vi "CRYPlot Result.vi"(7 "pGraph VI In":refnum<vi>, 8 "Graph Set?":bool, 9 "Flattened Property":string, 10 "New Rows In":i32[](array[numeric]), 11 "Old Rows In":i32[](array[numeric])) -> (2 "Curve Name":string[](array[string]), 3 "Selected Rows Out":i32[](array[numeric]))   [LabVIEW 2013]
uses:
  CRYWindow/DataView/Control/CRYResult Property.ctl
panel:
  in  "Result Property":T1={"Show Limits"=FALSE, "Show Yield"=FALSE, "Pass/Fail"=FALSE, "Notation"=0, "Digits"=0, "Precision"=0, "Hide Traling Zeros"=FALSE, "Show vertical scroll bar"=FALSE, "Show horizontal scroll bar"=FALSE, "True"="NO ELECTRICAL SIGNAL DETECTED!\nCheck wiring and connections.", "False"="NO ELECTRICAL SIGNAL DETECTED!\nCheck wiring and connections.", "Font Size"=0, "Overall/Optional"=0} {"Precision" items=["Digits of precision", "Significant digits"]}
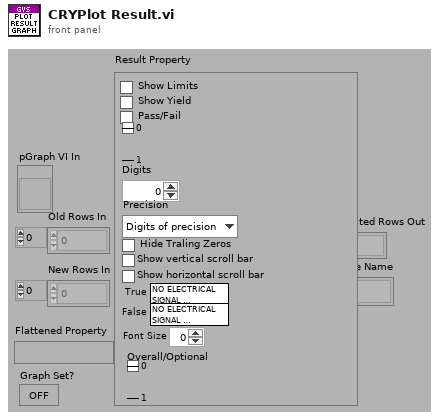
[diagram p1: front panel]
types:
  T1 = typedef "CRYResult Property.ctl" = cluster{"Show Limits":bool, "Show Yield":bool, "Pass/Fail":bool, "Notation":u16, "Digits":u16, "Precision":u16, "Hide Traling Zeros":bool, "Show vertical scroll bar":bool, "Show horizontal scroll bar":bool, "True":string, "False":string, "Font Size":u16, "Overall/Optional":u16}
  T2 = typedef "CRYResult Cluster.ctl" = cluster{"Name":string, "Margin":dbl, "unit":string, "Verdict":bool, "Limit":string, "Max/Min":string, "protected":bool, "Step No.":i32, "Test Info":string, "AutoProtect":bool}
  T3 = cluster{"left":i16, "top":i16, "right":i16, "bottom":i16}
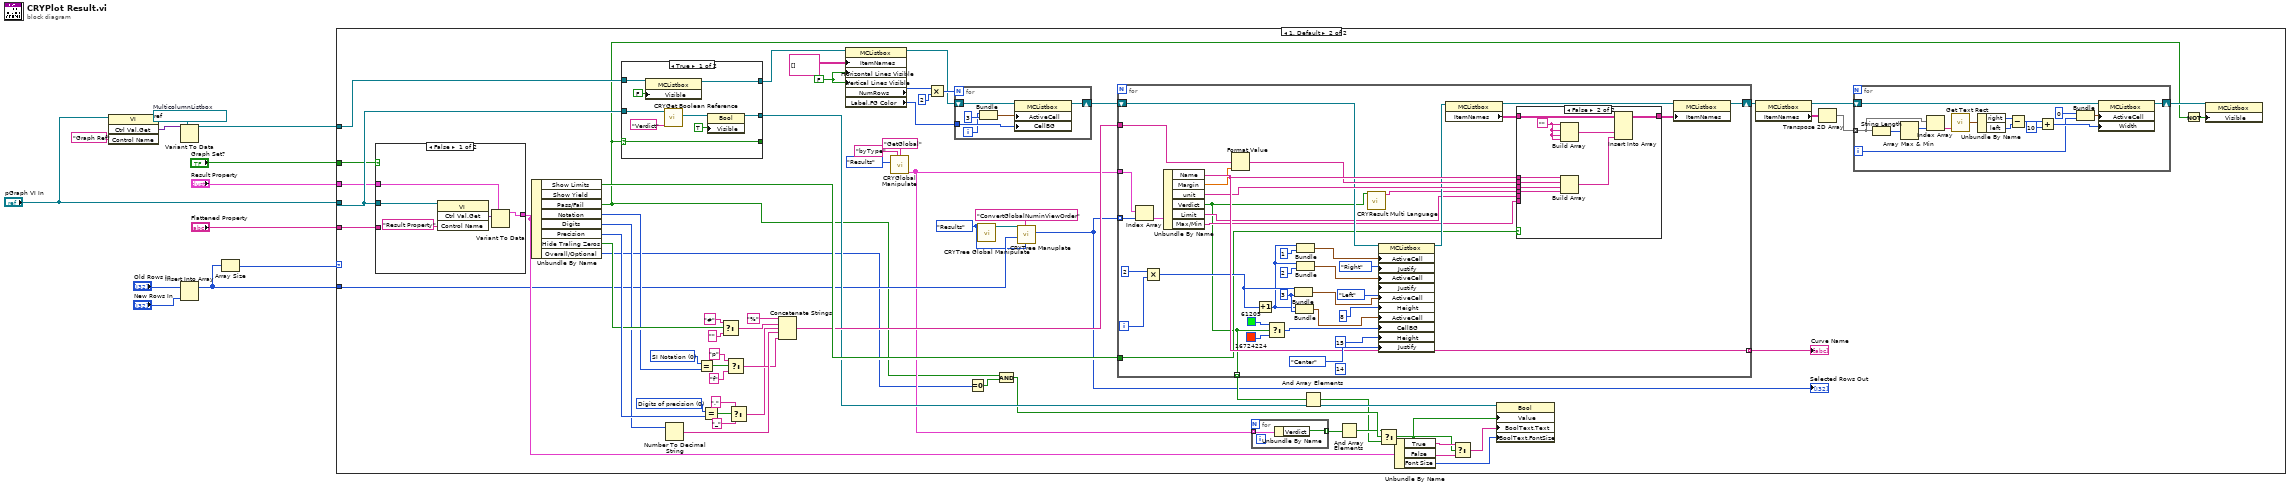
[diagram p0: block diagram]
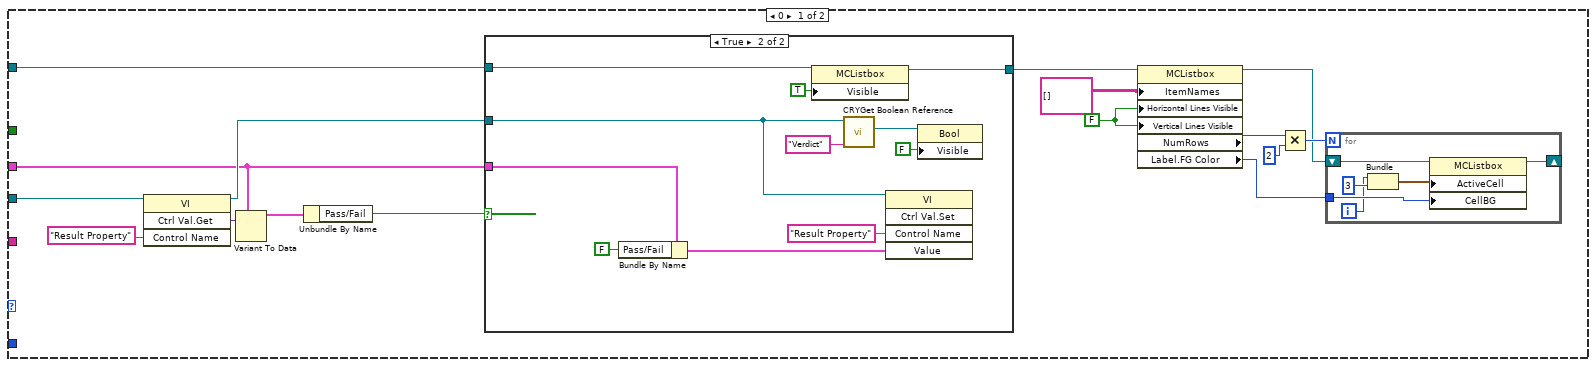
[diagram p2: hidden frame]
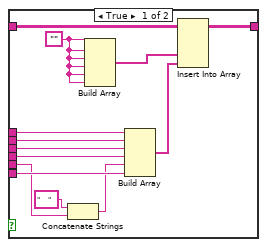
[diagram p4: hidden frame]
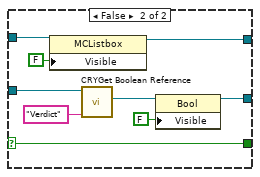
[diagram p5: hidden frame]
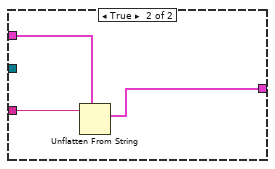
[diagram p6: hidden frame]
diagram:
  w7 = refnum<vi> refnum  # MulticolumnListbox
  n1 = invoke class="VI" method="Ctrl Val.Get"(reference="pGraph VI In", "Control Name"="Graph Ref") -> ("Get Control Value Variant"=w8:variant)  [unwired: 2 in, 3 out]
  n2 = Variant To Data(type=w7, Variant=w8) -> (data=w4:refnum<vi>)  [unwired: 1 in, 1 out]
  n3 = Insert Into Array(array="Old Rows In", new element="New Rows In") -> (w9:i32[])  [unwired: 1 in]
  n4 = Array Size(array=w9) -> (size(s)=w10:i32)
  n5 = case shown="1, Default" w10 {
    tunnel: w9 -> [_ w65]
    tunnel: "pGraph VI In" -> [w19 w63]
    tunnel: w4 -> [w16 w62]
    tunnel: "Graph Set?" -> [_ w61]
    tunnel: "Result Property" -> [w13 w60]
    tunnel: "Flattened Property" -> [_ w59]
    frame 0 {
      w26 = FALSE ("Visible Items:Horizontal Lines Visible")
      n6 = invoke class="VI" method="Ctrl Val.Get"(reference=w19, "Control Name"="Result Property") -> (reference out=w14:refnum<vi>, "Get Control Value Variant"=w20:variant)  [unwired: 2 in, 2 out]
      n7 = Variant To Data(type=w13, Variant=w20) -> (data=w18:T1)  [unwired: 1 in, 1 out]
      n8 = Unbundle By Name(w18) -> ("Pass/Fail"=w17:bool)
      n9 = case shown="True" w17 {
        tunnel: w16 -> [w29 w40]
        tunnel: w14 -> [_ w34]
        tunnel: [w29 w35] -> w15
        tunnel: w13 -> [_ w32]
        frame False {
        }
        frame True {
          n10 = Bundle By Name(cluster=w32, "Pass/Fail"=FALSE) -> (w30:T1)
          n11 = property class="MCListbox"(reference=w40, "Visible"=TRUE) -> (reference out=w35:refnum<vi>)  [unwired: 1 in, 1 out]
          n12 = call "CRYGet Boolean Reference.vi"("Label Name"="Verdict" ("Control Name"), "VI Refnum"=w34) -> ("Boolean Ref"=w37:refnum<vi>)  [unwired: 7 in, 2 out]
          n13 = invoke class="VI" method="Ctrl Val.Set"(reference=w34, "Control Name"="Result Property", "Value"=w30) -> ()  [unwired: 2 in, 5 out]
          n14 = property class="Bool"(reference=w37, "Visible"=FALSE) -> ()  [unwired: 1 in, 2 out]
        }
      }
      n15 = property class="MCListbox"(reference=w15, "ItemNames"=string[][] [] ("Item Names"), "Horizontal Lines Visible"=w26, "Vertical Lines Visible"=w26) -> (reference out=w22:refnum<vi>, "NumRows"=w27:u32, "Label.FG Color"=w25:u32)  [unwired: 1 in, 1 out]
      n16 = Multiply(x=w27, y=u32 2) -> (x*y=w24:u32)
      n17 = for {
        N: w24 -> [_]
        tunnel: w25 -> [w45]
        shift-right: [w41] -> _
        shift-left: w22 -> [w44]
        i -> [w42]
        n18 = Bundle(w42, 3) -> (w46:cluster{i32, i32})  [unwired: 1 out]
        n19 = property class="MCListbox"(reference=w44, "ActiveCell"=w46, "CellBG"=w45) -> (reference out=w41:refnum<vi>)  [unwired: 1 in, 1 out]
      }
    }
    frame 1, Default {
      w47 = enum16{"Curves", "Values", "Results", "WFM"}."Results" ("Type In")
      w83 = u16 0 items=["Digits of precision", "Significant digits"] ("Precision")
      w82 = u16 0 items=["SI Notation", "Floating point"] ("Notation")
      w105 = FALSE ("Visible Items:Horizontal Lines Visible")
      n20 = case shown="False" w61 {
        tunnel: w60 -> [w216 w220]
        tunnel: [w215 w219] -> w75
        tunnel: w63 -> [w214 _]
        tunnel: w59 -> [_ w221]
        frame False {
          n21 = invoke class="VI" method="Ctrl Val.Get"(reference=w214, "Control Name"="Result Property") -> ("Get Control Value Variant"=w217:variant)  [unwired: 2 in, 3 out]
          n22 = Variant To Data(type=w216, Variant=w217) -> (data=w215:T1)  [unwired: 1 in, 1 out]
        }
        frame True {
          n23 = Unflatten From String(type=w220, binary string=w221) -> (value=w219:T1)  [unwired: 3 in, 2 out]
        }
      }
      n24 = Unbundle By Name(w75) -> ("Show Limits"=w108:bool, "Pass/Fail"=w56:bool, "Notation"=w110:u16, "Digits"=w109:u16, "Precision"=w112:u16, "Hide Traling Zeros"=w111:bool, "Overall/Optional"=w53:u16)  [unwired: 1 out]
      n25 = case shown="True" w56 {
        selector: w56 -> [w204 w213]
        tunnel: [w204 w213] -> _
        tunnel: w62 -> [w203 w212]
        tunnel: w63 -> [w201 w210]
        tunnel: [w197 w206] -> w77
        tunnel: [w196 w205] -> w78
        frame True {
          n26 = property class="MCListbox"(reference=w203, "Visible"=FALSE) -> (reference out=w196:refnum<vi>)  [unwired: 1 in, 1 out]
          n27 = call "CRYGet Boolean Reference.vi"("Label Name"="Verdict" ("Control Name"), "VI Refnum"=w201) -> ("Boolean Ref"=w199:refnum<vi>)  [unwired: 7 in, 2 out]
          n28 = property class="Bool"(reference=w199, "Visible"=TRUE) -> (reference out=w197:refnum<vi>)  [unwired: 1 in, 1 out]
        }
        frame False {
          n29 = property class="MCListbox"(reference=w212, "Visible"=FALSE) -> (reference out=w205:refnum<vi>)  [unwired: 1 in, 1 out]
          n30 = call "CRYGet Boolean Reference.vi"("Label Name"="Verdict" ("Control Name"), "VI Refnum"=w210) -> ("Boolean Ref"=w208:refnum<vi>)  [unwired: 7 in, 2 out]
          n31 = property class="Bool"(reference=w208, "Visible"=FALSE) -> (reference out=w206:refnum<vi>)  [unwired: 1 in, 1 out]
        }
      }
      n32 = Number To Decimal String(number=w109) -> (decimal integer string=w96:string)  [unwired: 1 in]
      n33 = Equal?(x=w82, y=w110) -> (x = y?=w85:bool)
      n34 = Equal?(x=w83, y=w112) -> (x = y?=w91:bool)
      n35 = Select(t="#" ("format string"), s=w111, f="" ("format string")) -> (s? t:f=w90:string)
      n36 = Select(t="p" ("string"), s=w85, f="f" ("string")) -> (s? t:f=w95:string)
      n37 = Select(t=".", s=w91, f="_") -> (s? t:f=w92:string)
      n38 = Concatenate Strings("%" ("string"), w90, w92, w96, w95) -> (w97:string)
      n39 = property class="MCListbox"(reference=w78, "ItemNames"=string[][] [] ("Item Names"), "Horizontal Lines Visible"=w105, "Vertical Lines Visible"=w105) -> (reference out=w101:refnum<vi>, "NumRows"=w106:u32, "Label.FG Color"=w104:u32)  [unwired: 1 in, 1 out]
      n40 = call "CRYGlobal Manipulate.vi"("Type"=enum16{"Curves", "Values", "Results", "WFM"}."Results", "sOption"="byType", "sAction"="GetGlobal") -> ("Results Out"=w58:T2[])  [unwired: 6 in, 6 out]
      n41 = Multiply(x=w106, y=u32 2) -> (x*y=w103:u32)
      n42 = for {
        N: w103 -> [_]
        tunnel: w104 -> [w134]
        shift-right: [w130] -> w100
        shift-left: w101 -> [w133]
        i -> [w131]
        n43 = Bundle(w131, 3) -> (w135:cluster{i32, i32})  [unwired: 1 out]
        n44 = property class="MCListbox"(reference=w133, "ActiveCell"=w135, "CellBG"=w134) -> (reference out=w130:refnum<vi>)  [unwired: 1 in, 1 out]
      }
      n45 = Equal To 0?(x=w53) -> (x = 0?=w54:bool)
      n46 = call "CRYTree Global Manipulate.vi"("Type In"=w47) -> ("Tree/Curve Tree"=w48:refnum<vi>)  [unwired: 7 in, 3 out]
      n47 = Compound Arithmetic op=AND(w56, w54) -> (w55:bool)
      n48 = call "CRYTree Manuplate.vi"("Type"=w47, "sAction"="ConvertGlobalNuminViewOrder", "nData"=w65, "Tree in"=w48) -> ("nData Out"=w64:i32[])  [unwired: 4 in, 3 out]
      "Selected Rows Out" <- w64
      n49 = for {
        tunnel: w58 -> [w172]
        tunnel: w64 -> [w161] mode=indexing
        tunnel: [w157] -> w99 mode=indexing
        shift-right: [w142] -> w79
        shift-left: w100 -> [w146]
        tunnel: w97 -> [w141]
        tunnel: w108 -> [w140]
        tunnel: [w137] -> w76 mode=indexing
        i -> [w167]
        (unwired) u32 14 ("Active Cell:Cell Font:Size")
        w165 = 3
        n50 = Index Array(array=w172, index=w161) -> (element=w173:T2)
        n51 = Multiply(x=2, y=w167) -> (x*y=w151:i32)
        n52 = Unbundle By Name(w173) -> ("Name"=w157:string, "Margin"=w156:dbl, "unit"=w154:string, "Verdict"=w137:bool, "Limit"=w139:string, "Max/Min"=w138:string)
        n53 = Format Value(format string=w141, value (0)=w156) -> (output string=w155:string)  [unwired: 1 out]
        n54 = Increment(x=w151) -> (x+1=w143:i32)
        n55 = Select(t=u32 61205, s=w137, f=u32 16724224) -> (s? t:f=w168:u32)
        n56 = Bundle(w151, w165) -> (w164:cluster{i32, i32})  [unwired: 1 out]
        n57 = Bundle(w143, w165) -> (w171:cluster{i32, i32})  [unwired: 1 out]
        n58 = Bundle(w143, 1) -> (w148:cluster{i32, i32})  [unwired: 1 out]
        n59 = Bundle(w143, 2) -> (w147:cluster{i32, i32})  [unwired: 1 out]
        n60 = call "CRYResult Multi Language.vi"("Verdict"=w137) -> ("ASCII out"=w136:string)  [unwired: 10 in]
        n61 = property class="MCListbox"(reference=w146, "ActiveCell"=w148, "Justify"=enum16{"Left", "Center", "Right"}."Right" ("Active Cell:Cell Justification"), "ActiveCell"=w147, "Justify"=enum16{"Left", "Center", "Right"}."Left" ("Active Cell:Cell Justification"), "ActiveCell"=w164, "Height"=u32 8 ("Active Cell:Cell Size:Height"), "ActiveCell"=w171, "CellBG"=w168, "Height"=u32 15 ("Active Cell:Cell Size:Height"), "Justify"=enum16{"Left", "Center", "Right"}."Center" ("Active Cell:Cell Justification")) -> (reference out=w144:refnum<vi>)  [unwired: 1 in, 1 out]
        n62 = property class="MCListbox"(reference=w144) -> (reference out=w145:refnum<vi>, "ItemNames"=w160:string[][])  [unwired: 1 in, 1 out]
        n63 = case shown="False" w140 {
          tunnel: w160 -> [w186 w195]
          tunnel: [w183 w192] -> w159
          tunnel: w157 -> [w182 w191]
          tunnel: w155 -> [w181 w189]
          tunnel: w136 -> [w180 w188]
          tunnel: w154 -> [w179 w187]
          tunnel: w139 -> [w175 _]
          tunnel: w138 -> [w177 _]
          frame True {
            w178 = ""
            n64 = Concatenate Strings("    " ("string"), w175) -> (w174:string)
            n65 = Build Array(w178, w178, w178, w178, w178, w178) -> (w185:string[])
            n66 = Build Array(w182, w181, w179, w180, w174, w177) -> (w184:string[])
            n67 = Insert Into Array(array=w186, new element #1=w185, new element #2=w184) -> (w183:string[][])  [unwired: 2 in]
          }
          frame False {
            w190 = ""
            n68 = Build Array(w190, w190, w190, w190) -> (w194:string[])
            n69 = Build Array(w191, w189, w187, w188) -> (w193:string[])
            n70 = Insert Into Array(array=w195, new element #1=w194, new element #2=w193) -> (w192:string[][])  [unwired: 2 in]
          }
        }
        n71 = property class="MCListbox"(reference=w145, "ItemNames"=w159) -> (reference out=w142:refnum<vi>)  [unwired: 1 in, 1 out]
      }
      "Curve Name" <- w99
      n72 = for {
        tunnel: w58 -> [w114] mode=indexing
        tunnel: [w113] -> w57 mode=indexing
        n73 = Unbundle By Name(w114) -> ("Verdict"=w113:bool)
      }
      n74 = And Array Elements(Boolean array=w76) -> (logical AND=w51:bool)
      n75 = And Array Elements(Boolean array=w57) -> (logical AND=w52:bool)
      n76 = Select(t=w52, s=w55, f=w51) -> (s? t:f=w50:bool)
      n77 = Unbundle By Name(w75) -> ("True"=w74:string, "False"=w73:string, "Font Size"=w71:u16)
      n78 = Select(t=w74, s=w50, f=w73) -> (s? t:f=w72:string)
      n79 = property class="Bool"(reference=w77, "Value"=w50, "BoolText.Text"=w72, "BoolText.FontSize"=w71) -> ()  [unwired: 1 in, 2 out]
      n80 = property class="MCListbox"(reference=w79) -> (reference out=w80:refnum<vi>, "ItemNames"=w98:string[][])  [unwired: 1 in, 1 out]
      n81 = Transpose 2D Array(2D array=w98) -> (transposed array=w81:string[][])
      n82 = for {
        tunnel: w81 -> [w118] mode=indexing
        shift-right: [w115] -> w70
        shift-left: w80 -> [w116]
        i -> [w117]
        n83 = String Length(string=w118) -> (length=w119:i32[])
        n84 = Array Max & Min(array=w119) -> (max index (indices)=w129:i32)  [unwired: 3 out]
        n85 = Index Array(array=w118, index=w129) -> (element=w124:string)
        n86 = call <vilib>:"Get Text Rect.vi"("text"=w124) -> ("rect"=w123:T3)  [unwired: 5 in, 3 out]
        n87 = Unbundle By Name(w123) -> ("right"=w127:i16, "left"=w126:i16)
        n88 = Subtract(x=w127, y=w126) -> (x-y=w128:i16)
        n89 = Add(x=w128, y=i16 10) -> (x+y=w120:i16)
        n90 = Bundle("Numeric"=i16 0, w117) -> (w122:cluster{"Numeric":i16, i32})  [unwired: 1 out]
        n91 = property class="MCListbox"(reference=w116, "ActiveCell"=w122, "Width"=w120) -> (reference out=w115:refnum<vi>)  [unwired: 1 in, 1 out]
      }
      n92 = Not(x=w56) -> (.not. x?=w69:bool)
      n93 = property class="MCListbox"(reference=w70, "Visible"=w69) -> ()  [unwired: 1 in, 2 out]
    }
  }
